vi "RaiseElevator-C.vi"(11 "Params":string[][](array[string])) -> ()   [LabVIEW 2018]
uses:
  Framework/Robot Global Data.vi
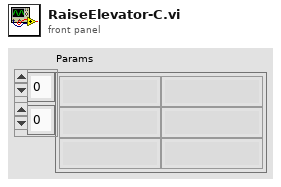
[diagram p1: front panel]
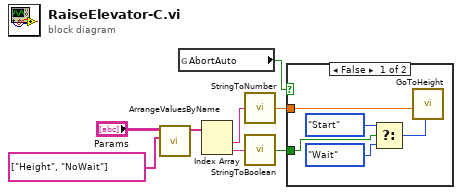
[diagram p0: block diagram]
diagram:
  n1 = call "ArrangeValuesByName.vi"("Names"=string[] ["Height", "NoWait"], "Names/Values in"="Params") -> ("Values Out"=w3:string[])  [unwired: 9 in]
  n2 = global read "Robot Global Data.vi" "AbortAuto"() -> (w8:bool)
  n3 = Index Array(array=w3) -> (element #1=w2:string, element #2=w1:string)  [unwired: 2 in]
  n4 = call "StringToNumber.vi"("String"=w2) -> ("Output"=w7:dbl)
  n5 = call "StringToBoolean.vi"("String"=w1) -> ("Output"=w6:bool)
  n6 = case shown="False" w8 {
    tunnel: w6 -> [w11 _]
    tunnel: w7 -> [w10 _]
    frame False {
      n7 = Select(t=enum16{"Start", "Wait"}."Start", s=w11, f=enum16{"Start", "Wait"}."Wait" ("Synchronication")) -> (s? t:f=w9:enum16{"Start", "Wait"})
      n8 = call "GoToHeight.vi"("Synchronization"=w9, "Setpoint"=w10) -> ()  [unwired: 9 in, 1 out]
    }
    frame True {
    }
  }
